vi "TraverseDoAllChannels.vi"(0 "Current Pulses positions for all channels":dbl[](array[numeric]), 1 "Current Pos In Eng units of all channels":dbl[](array[numeric]) format="%.2f", 2 "Counters Reset?":bool, 5 "Backlash Compensation?":bool, 7 "Home":T1, 9 "Mode":T5, 11 "Position Steps":dbl[][](array[numeric]) format="%.2f", 12 "Matched Configurations all Channels In":T2[](array[typedef]) {"Static Drive Configuration"."Indexer Mode  (FSA)" items=["Incremental", "Absolute"]; "Static Drive Configuration"."Buffer at Stop (SSH)" items=["Clear buffer", "Save and Continue"]; "Static Drive Configuration"."Buffer at Limit (SSG)" items=["Clear buffer", "Save and Continue"]; "Static Drive Configuration"."RS232 Echo Control (SSA)" items=["Echo ON", "Echo OFF"]; "Static Drive Configuration"."Reference edge of Home (OSH)" items=["CW", "CCW"]; "Static Drive Configuration"."Encoder Z for Home (OSD)" items=["Don't use", "Enable"]; "Static Drive Configuration"."Home Switch Sense (OSC)" items=["Normally Open", "Normally Closed"]; "Static Drive Configuration"."Home Position (OSB)" items=["Anywhere in Switch", "Edge of Switch"]; "Static Drive Configuration"."Limit Switch Sense (OSA)" items=["Normally Closed", "Normally Open"]; "Static Drive Configuration"."Limit Disable (LD)" items=["Both Enabled", "CW Disabled", "CCW Disabled", "Both Disabled"]; "Static Drive Configuration"."Stall Detect (FSH)" items=["Disable", "Enable"]; "Static Drive Configuration"."OP2 in Deadband (FSG)" items=["Don't Use", "ACTIVATE"]; "Static Drive Configuration"."Stop on Trigger 3 (FSF)" items=["Ignore", "STOP!"]; "Static Drive Configuration"."Activate OP1 on stall (FSE)" items=["Do not Activate", "ACTIVATE!"]; "Static Drive Configuration"."Stop on Stall (FSD)" items=["Continue", "STOP"]; "Static Drive Configuration"."Position Maintenance (FSC)" items=["Disabled", "Enabled"]; "Static Drive Configuration"."Step Mode  (FSB)" items=["Motor", "Encoder"]; "Static Drive Configuration"."Encoder Resolution (ER)" min=1 max=50000; "Static Drive Configuration"."Dead Band Window (DW)" min=0 max=999999999; "Static Drive Configuration"."Dead Band (DB)" min=0 max=999999999; "Static Drive Configuration"."Correction Gain % (CG)" items=["n/a", "12.5", "25", "37.5", "50", "62.5", "75", "87.5", "100"]; "Channel Properties"."Current Pos" format="%.2f"; "Channel Properties"."Backlash/Eng units" format="%.2f"; "Channel Properties"."Pulses/rev" format="%.2f"; "Channel Properties"."Pos Tolerance" format="%.2f"; "Channel Properties"."Pulses/unit" format="%.2f"; "Channel Properties"."Acc. Min" format="%.2f"; "Channel Properties"."Acc. Max" format="%.2f"; "Channel Properties"."Vel. Min" format="%.2f"; "Channel Properties"."Vel. Max" format="%.2f"; "Channel Properties"."Acc. Default" format="%.2f"; "Channel Properties"."Vel. Default" format="%.2f"}, 13 "Last Part of Move?":bool, 14 "Traverse Name":string="EnFlo Tunnel") -> (4 "Achieved Pos In Eng units of all channels":dbl[](array[numeric]) format="%.2f", 6 "Current Pulses positions for all channels Out":dbl[](array[numeric]), 10 "Error String":string, 15 "Matched Configurations Out":T2[](array[typedef]) {"Static Drive Configuration"."Indexer Mode  (FSA)" items=["Incremental", "Absolute"]; "Static Drive Configuration"."Buffer at Stop (SSH)" items=["Clear buffer", "Save and Continue"]; "Static Drive Configuration"."Buffer at Limit (SSG)" items=["Clear buffer", "Save and Continue"]; "Static Drive Configuration"."RS232 Echo Control (SSA)" items=["Echo ON", "Echo OFF"]; "Static Drive Configuration"."Reference edge of Home (OSH)" items=["CW", "CCW"]; "Static Drive Configuration"."Encoder Z for Home (OSD)" items=["Don't use", "Enable"]; "Static Drive Configuration"."Home Switch Sense (OSC)" items=["Normally Open", "Normally Closed"]; "Static Drive Configuration"."Home Position (OSB)" items=["Anywhere in Switch", "Edge of Switch"]; "Static Drive Configuration"."Limit Switch Sense (OSA)" items=["Normally Closed", "Normally Open"]; "Static Drive Configuration"."Limit Disable (LD)" items=["Both Enabled", "CW Disabled", "CCW Disabled", "Both Disabled"]; "Static Drive Configuration"."Stall Detect (FSH)" items=["Disable", "Enable"]; "Static Drive Configuration"."OP2 in Deadband (FSG)" items=["Don't Use", "ACTIVATE"]; "Static Drive Configuration"."Stop on Trigger 3 (FSF)" items=["Ignore", "STOP!"]; "Static Drive Configuration"."Activate OP1 on stall (FSE)" items=["Do not Activate", "ACTIVATE!"]; "Static Drive Configuration"."Stop on Stall (FSD)" items=["Continue", "STOP"]; "Static Drive Configuration"."Position Maintenance (FSC)" items=["Disabled", "Enabled"]; "Static Drive Configuration"."Step Mode  (FSB)" items=["Motor", "Encoder"]; "Static Drive Configuration"."Encoder Resolution (ER)" min=1 max=50000; "Static Drive Configuration"."Dead Band Window (DW)" min=0 max=999999999; "Static Drive Configuration"."Dead Band (DB)" min=0 max=999999999; "Static Drive Configuration"."Correction Gain % (CG)" items=["n/a", "12.5", "25", "37.5", "50", "62.5", "75", "87.5", "100"]; "Channel Properties"."Current Pos" format="%.2f"; "Channel Properties"."Backlash/Eng units" format="%.2f"; "Channel Properties"."Pulses/rev" format="%.2f"; "Channel Properties"."Pos Tolerance" format="%.2f"; "Channel Properties"."Pulses/unit" format="%.2f"; "Channel Properties"."Acc. Min" format="%.2f"; "Channel Properties"."Acc. Max" format="%.2f"; "Channel Properties"."Vel. Min" format="%.2f"; "Channel Properties"."Vel. Max" format="%.2f"; "Channel Properties"."Acc. Default" format="%.2f"; "Channel Properties"."Vel. Default" format="%.2f"})   [LabVIEW 2014]
uses:
  Anemometry/Anemometry Sub Vis/Gen Trav/Trav_mode.ctl
  ~subVIs/AxisConfigCluster.ctl
  ~subVIs/DriveProperties.ctl
  ~subVIs/DriveStaticConfig.ctl
  Anemometry/Anemometry Sub Vis/Controls/Home.ctl
  ~subVIs/DriveGotoCluster.ctl
  ~subVIs/DriveConfigGlobal.vi
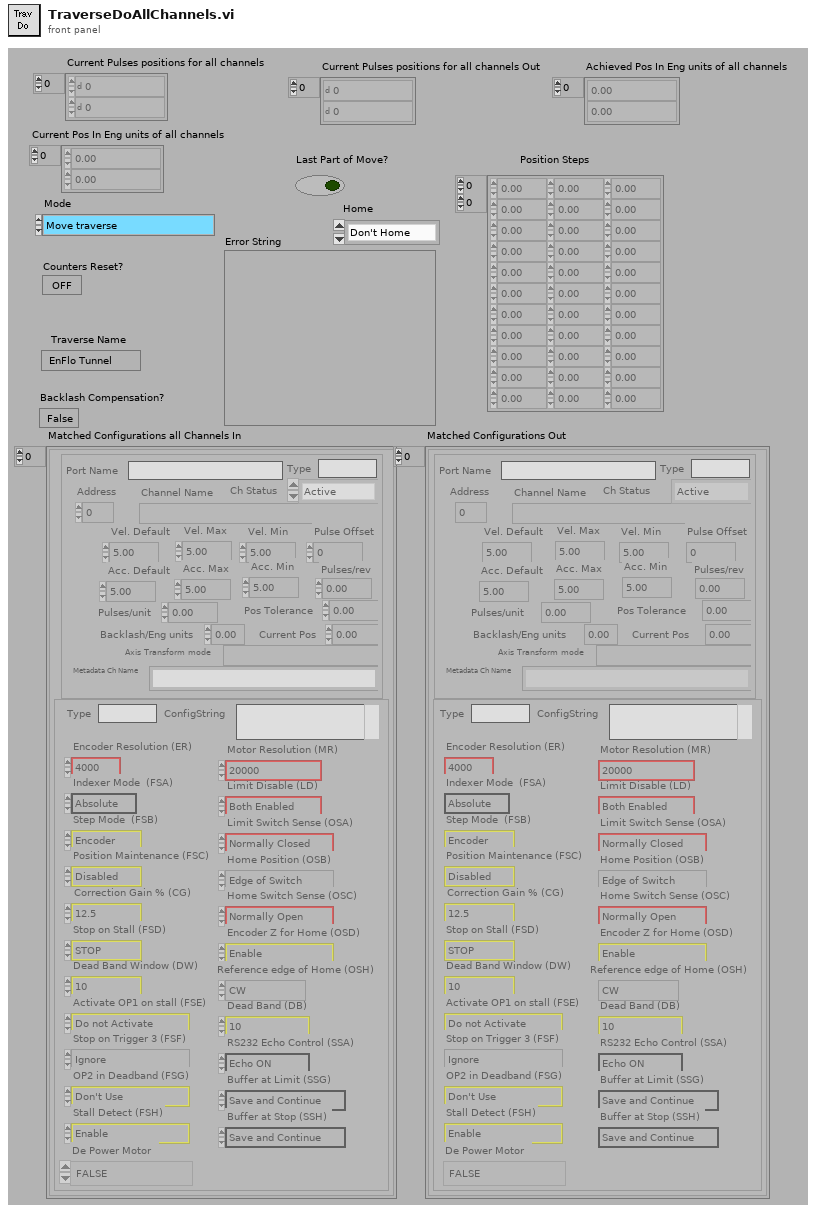
[diagram p1: front panel]
types:
  T1 = typedef "Home.ctl" = enum16{"Don't Home", "Home  +X", "Home  -X", "Home  +Y", "Home  -Y", "Home  +Z", "Home  -Z"}
  T2 = typedef "AxisConfigCluster.ctl" = cluster{"Channel Properties":T3, "Static Drive Configuration":T4}
  T3 = typedef "DriveProperties.ctl" = cluster{"Channel Name":string, "Vel. Default":dbl, "Acc. Default":dbl, "Vel. Max":dbl, "Vel. Min":dbl, "Acc. Max":dbl, "Acc. Min":dbl, "Pulses/unit":dbl, "Address":u8, "Pulse Offset":i32, "Pos Tolerance":dbl, "Pulses/rev":dbl, "Backlash/Eng units":dbl, "Current Pos":dbl, "Ch Status":enum16{"Active", "Offline", "Simulate"}, "Port Name":string, "Axis Transform mode":string, "Metadata Ch Name":string, "Type":string}
  T4 = typedef "DriveStaticConfig.ctl" = cluster{"Correction Gain % (CG)":u16, "Dead Band (DB)":i32, "Dead Band Window (DW)":i32, "Encoder Resolution (ER)":i32, "Step Mode  (FSB)":u16, "Position Maintenance (FSC)":u16, "Stop on Stall (FSD)":u16, "Activate OP1 on stall (FSE)":u16, "Stop on Trigger 3 (FSF)":u16, "OP2 in Deadband (FSG)":u16, "Stall Detect (FSH)":u16, "Limit Disable (LD)":u16, "Motor Resolution (MR)":enum16{"200", "400", "1000", "2000", "4000", "5000", "10000", "12800", "18000", "20000", "21600", "25000", "25400", "25600", "36000", "50000", "278528", "425984", "507904", "614400", "655360", "819200", "1024000"}, "Limit Switch Sense (OSA)":u16, "Home Position (OSB)":u16, "Home Switch Sense (OSC)":u16, "Encoder Z for Home (OSD)":u16, "Reference edge of Home (OSH)":u16, "RS232 Echo Control (SSA)":u16, "Buffer at Limit (SSG)":u16, "Buffer at Stop (SSH)":u16, "Indexer Mode  (FSA)":u16, "Type":string, "ConfigString":string, "De Power Motor":enum16{"TRUE", "FALSE"}}
  T5 = typedef "Trav_mode.ctl" = enum16{"Move traverse", "Read traverse position", "Teach Position"}
  T6 = enum16{"Load setup from excel file", "Save setup to excel file"}
  T7 = typedef "DriveGotoCluster.ctl" = cluster{"Channel name":string, "Go To Position":dbl}
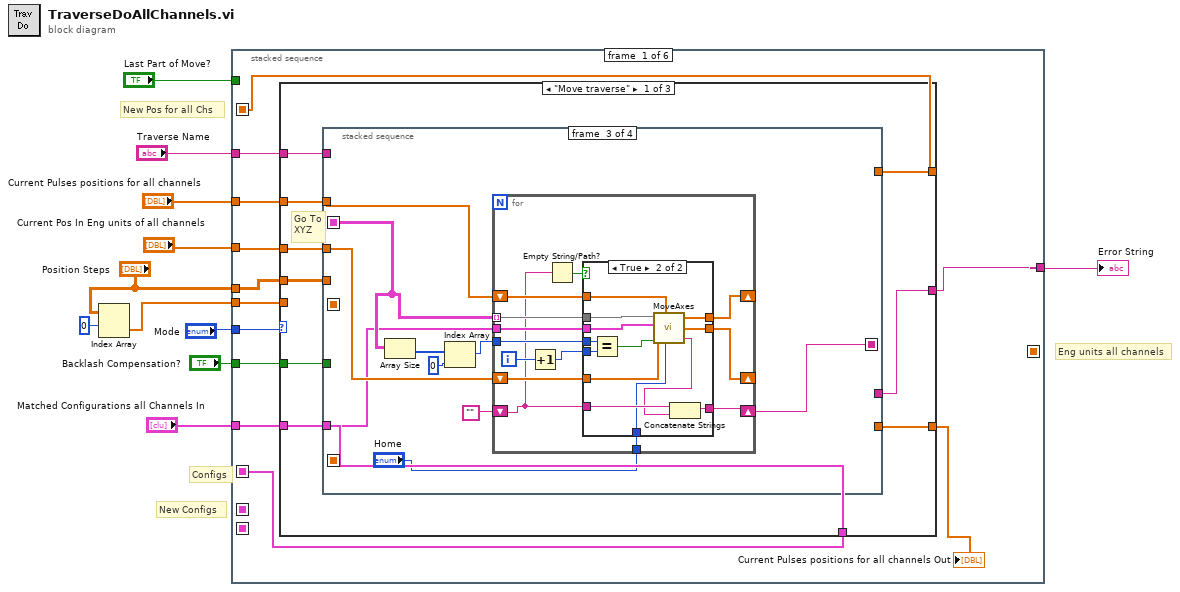
[diagram p0: block diagram]
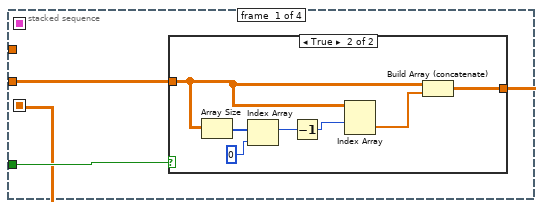
[diagram p2: hidden frame]
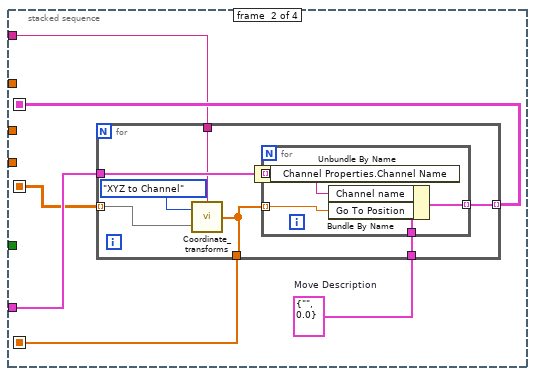
[diagram p4: hidden frame]
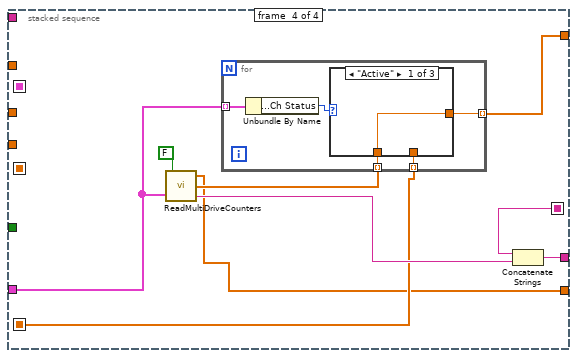
[diagram p6: hidden frame]
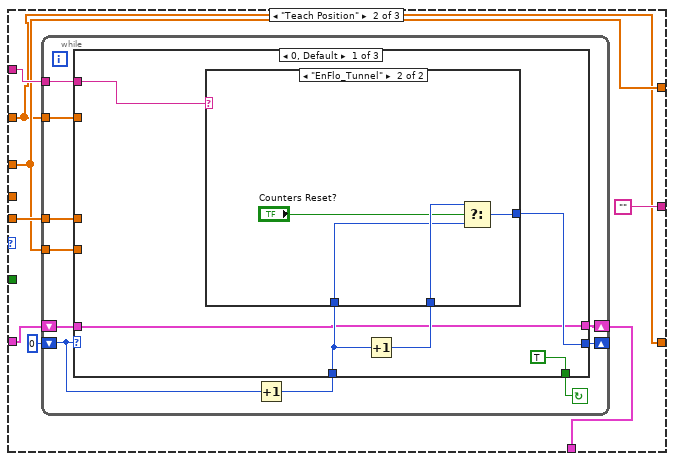
[diagram p9: hidden frame]
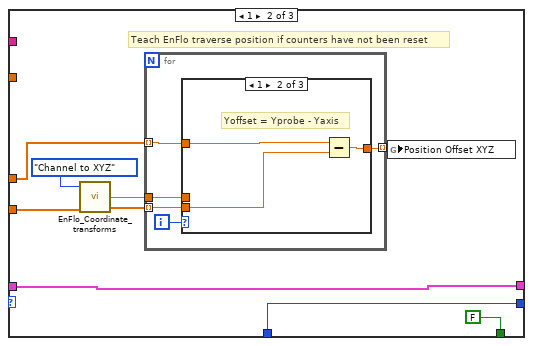
[diagram p11: hidden frame]
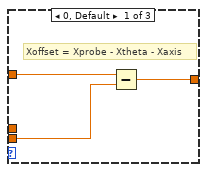
[diagram p12: hidden frame]
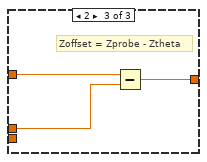
[diagram p13: hidden frame]
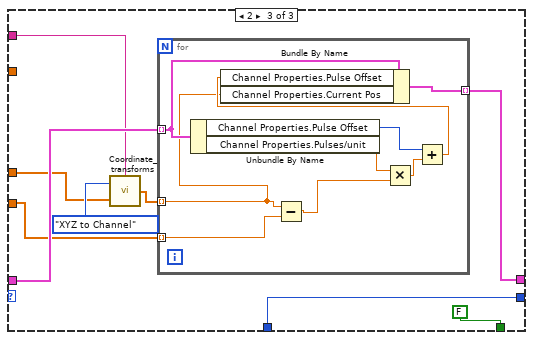
[diagram p14: hidden frame]
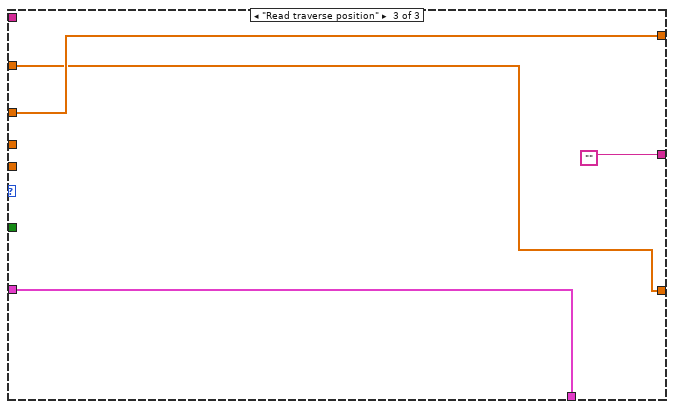
[diagram p15: hidden frame]
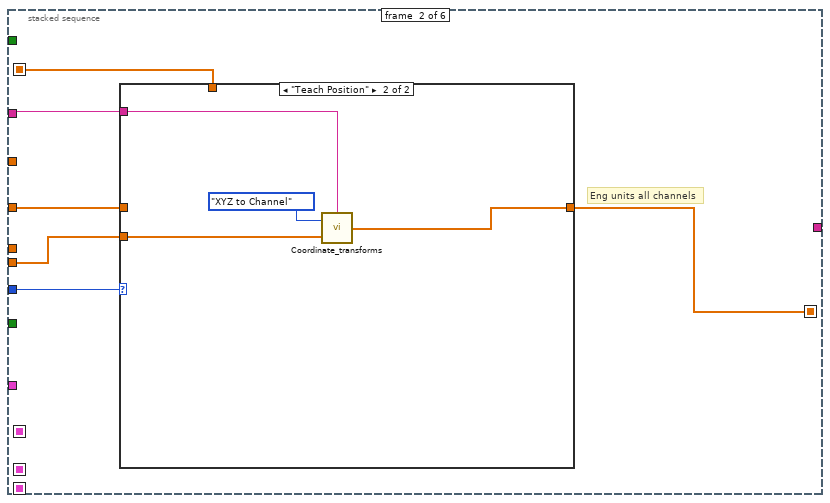
[diagram p16: hidden frame]
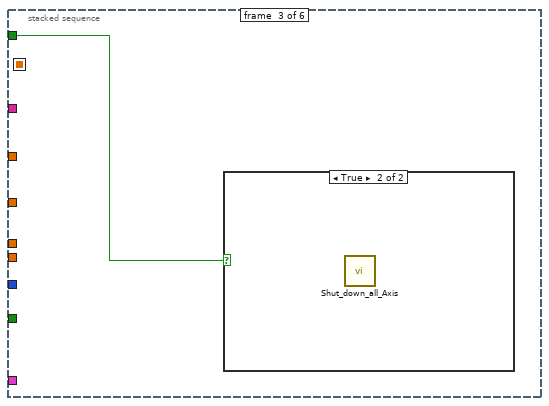
[diagram p18: hidden frame]
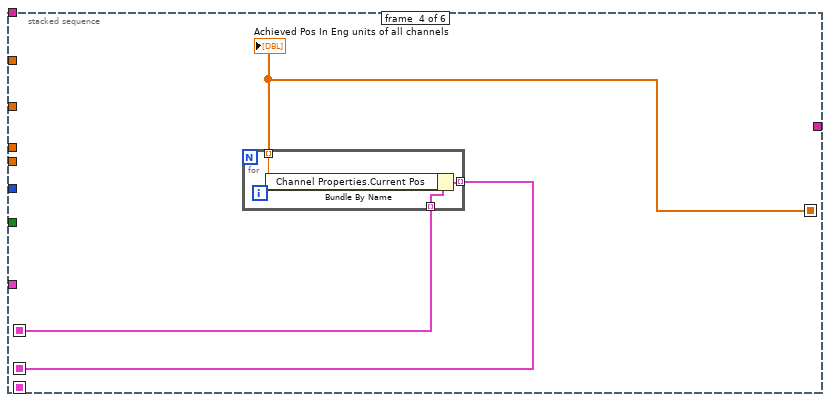
[diagram p20: hidden frame]
diagram:
  # "New Pos for all Chs"
  # "Eng units all channels"
  # "New Configs"
  # "Configs"
  n1 = Index Array(array="Position Steps", index (row)=0 ("Index")) -> (element=w2:dbl[])  [unwired: 1 in]
  n2 = stacked-sequence {
    seq-local: [_ w195 _ _ _ _] -> [_ _ _ w204 _ _]
    seq-local: [w22 _ _ _ _ _] -> [_ _ _ w206 _ _]
    seq-local: [_ _ _ w205 _ _] -> [_ _ _ _ w213 _]
    seq-local: [w13 _ _ _ _ _] -> [_ w192 _ _ _ _]
    seq-local: [_ _ _ _ w211 _] -> [_ _ _ _ _ w220]
    tunnel: "Mode" -> [w23 w196 _ _ _ w221]
    tunnel: "Current Pos In Eng units of all channels" -> [w20 w197 _ _ _ _]
    tunnel: "Matched Configurations all Channels In" -> [w21 _ _ _ _ _]
    tunnel: "Current Pulses positions for all channels" -> [w19 _ _ _ _ _]
    tunnel: [w18 _ _ _ _ _] -> w7
    tunnel: "Traverse Name" -> [w17 w194 _ _ w212 w219]
    tunnel: "Position Steps" -> [w16 _ _ _ _ _]
    tunnel: "Backlash Compensation?" -> [w15 _ _ _ _ _]
    tunnel: w2 -> [w14 w193 _ _ _ _]
    tunnel: "Last Part of Move?" -> [_ _ w203 _ w210 _]
    frame #0 {
      n3 = case shown="\"Move traverse\"" w23 {
        tunnel: [w32 w122 w191] -> w22
        tunnel: w21 -> [w32 w123 w191]
        tunnel: w20 -> [w30 w119 w189]
        tunnel: w19 -> [w31 w118 w188]
        tunnel: [w29 "" ""] -> w18
        tunnel: w17 -> [w27 w124 _]
        tunnel: w16 -> [w28 _ _]
        tunnel: w15 -> [w26 _ _]
        tunnel: w14 -> [_ w120 _]
        tunnel: [w25 w119 w189] -> w13
        tunnel: [w24 w118 w188] -> w12
        frame "Move traverse" {
          # "Go To\nXYZ"
          n4 = stacked-sequence {
            seq-local: [_ w47 _ _] -> [_ _ w65 _]
            seq-local: [w34 _ _ _] -> [_ w46 _ _]
            seq-local: [_ _ w63 _] -> [_ _ _ w108]
            seq-local: [_ w44 _ _] -> [_ _ _ w102]
            tunnel: w32 -> [_ w48 w64 w105]
            tunnel: w31 -> [_ _ w71 _]
            tunnel: w30 -> [_ _ w70 _]
            tunnel: [_ _ _ w106] -> w29
            tunnel: w28 -> [w33 _ _ _]
            tunnel: w27 -> [_ w45 _ _]
            tunnel: w26 -> [w35 _ _ _]
            tunnel: [_ _ _ w104] -> w25
            tunnel: [_ _ _ w101] -> w24
            frame #0 {
              n5 = case shown="True" w35 {
                tunnel: w33 -> [w36 w38]
                tunnel: [w36 w37] -> w34
                frame False {
                }
                frame True {
                  n6 = Array Size(array=w38) -> (size(s)=w43:i32[])
                  n7 = Index Array(array=w43, index=0 ("Index")) -> (element=w41:i32)
                  n8 = Decrement(x=w41) -> (x-1=w40:i32)
                  n9 = Index Array(array=w38, index (row)=w40) -> (element=w39:dbl[])  [unwired: 1 in]
                  n10 = Build Array (concatenate)(w38, w39) -> (w37:dbl[][])
                }
              }
            }
            frame #1 {
              w49 = T7 {"Channel name"="", "Go To Position"=0.0}  # Move Description
              n11 = for {
                tunnel: w49 -> [w56]
                tunnel: w48 -> [w55]
                tunnel: [w54] -> w47 mode=indexing
                tunnel: w46 -> [w51] mode=indexing
                tunnel: w45 -> [w52]
                tunnel: [w50] -> w44
                n12 = call "Coordinate_transforms.vi"("Traverse Name"=w52, "Input"=w51, "Mode"=enum16{"XYZ to Channel", "Channel to XYZ"}."XYZ to Channel") -> ("Output"=w50:dbl[])
                n13 = for {
                  tunnel: w50 -> [w61] mode=indexing
                  tunnel: [w60] -> w54 mode=indexing
                  tunnel: w55 -> [w58] mode=indexing
                  tunnel: w56 -> [w57]
                  n14 = Unbundle By Name(w58) -> ("Channel Properties.Channel Name"=w59:string)
                  n15 = Bundle By Name(cluster=w57, "Channel name"=w59, "Go To Position"=w61) -> (w60:T7)
                }
              }
            }
            frame #2 {
              n16 = Array Size(array=w65) -> (size(s)=w68:i32[])
              n17 = Index Array(array=w68, index=0 ("Index")) -> (element=w66:i32)
              n18 = for {
                tunnel: w65 -> [w84] mode=indexing
                tunnel: w64 -> [w83]
                shift-right: [w80] -> _
                shift-left: w71 -> [w79]
                shift-right: [w81] -> _
                shift-left: w70 -> [w82]
                tunnel: w66 -> [w76]
                shift-right: [w75] -> w63
                shift-left: "" -> [w74]
                tunnel: "Home" -> [w72]
                i -> [w78]
                n19 = Increment(x=w78) -> (x+1=w77:i32)
                n20 = Empty String/Path?(string/path=w74) -> (empty?=w73:bool)
                n21 = case shown="True" w73 {
                  tunnel: w84 -> [_ w100]
                  tunnel: w83 -> [_ w99]
                  tunnel: w82 -> [w86 w98]
                  tunnel: [w86 w97] -> w81
                  tunnel: [w87 w96] -> w80
                  tunnel: w79 -> [w87 w95]
                  tunnel: w77 -> [_ w94]
                  tunnel: w76 -> [_ w93]
                  tunnel: [w85 w90] -> w75
                  tunnel: w74 -> [w85 w92]
                  tunnel: w72 -> [_ w88]
                  frame False {
                  }
                  frame True {
                    n22 = Equal?(x=w93, y=w94) -> (x = y?=w89:bool)
                    n23 = call "MoveAxes.vi"("GoTo Array (Eng units all channels)"=w100, "Current Pulses In"=w95, "Matched Configurations"=w99, "Current Pos In"=w98, "Home"=w88, "Final move"=w89) -> ("Current Pulses Out"=w96:dbl[], "Current Pos Out"=w97:dbl[], "Error String"=w91:string)
                    n24 = Concatenate Strings(w92, w91) -> (w90:string)
                  }
                }
              }
            }
            frame #3 {
              n25 = call "ReadMultiDriveCounters.vi"("Recheck if Moved?"=FALSE, "Matched Configurations"=w105) -> ("Pulses"=w101:dbl[], "Eng units"=w103:dbl[], "Error String"=w107:string)
              n26 = for {
                tunnel: w105 -> [w114] mode=indexing
                tunnel: [w112] -> w104 mode=indexing
                tunnel: w103 -> [w111] mode=indexing
                tunnel: w102 -> [w110] mode=indexing
                n27 = Unbundle By Name(w114) -> ("Channel Properties.Ch Status"=w113:enum16{"Active", "Offline", "Simulate"})
                n28 = case shown="\"Active\"" w113 {
                  tunnel: [w115 w116 w117] -> w112
                  tunnel: w111 -> [w115 _ w117]
                  tunnel: w110 -> [_ w116 _]
                  frame "Active" {
                  }
                  frame "Simulate" {
                  }
                  frame "Offline" {
                  }
                }
              }
              n29 = Concatenate Strings(w108, w107) -> (w106:string)
            }
          }
        }
        frame "Teach Position" {
          n30 = while {
            tunnel: w120 -> [w126]
            shift-left: w123 -> [w128]
            shift-right: [w127] -> w122
            tunnel: w119 -> [w129]
            tunnel: w118 -> [w130]
            tunnel: w124 -> [w131]
            shift-left: 0 -> [w135]
            shift-right: [w132] -> _
            stop <- w134 continue-if-true
            n31 = Increment(x=w135) -> (x+1=w133:i32)
            n32 = case shown="0, Default" w135 {
              tunnel: [TRUE FALSE FALSE] -> w134
              tunnel: w133 -> [w138 w149 w178]
              tunnel: [w139 w149 w178] -> w132
              tunnel: w131 -> [w140 _ w171]
              tunnel: w130 -> [_ _ _]
              tunnel: w129 -> [_ w150 w172]
              tunnel: w128 -> [w136 w148 w176]
              tunnel: [w136 w148 w175] -> w127
              tunnel: w126 -> [_ w147 w170]
              frame 0, Default {
                n33 = Increment(x=w138) -> (x+1=w137:i32)
                n34 = case shown="\"EnFlo_Tunnel\"" w140 {
                  tunnel: [w142 w146] -> w139
                  tunnel: w138 -> [_ w144]
                  tunnel: w137 -> [w142 w145]
                  frame "A_Tunnel", Default {
                  }
                  frame "EnFlo_Tunnel" {
                    n35 = Select(t=w145, s="Counters Reset?", f=w144) -> (s? t:f=w146:i32)
                  }
                }
              }
              frame 1 {
                # "Teach EnFlo traverse position if counters have not been reset"
                n36 = call "EnFlo_Coordinate_transforms.vi"("Input"=w150, "Mode"=enum16{"XYZ to Channel", "Channel to XYZ"}."Channel to XYZ") -> ("Output"=w153:dbl[], "Z theta"=w152:dbl)  [unwired: 2 out]
                n37 = for {
                  tunnel: w147 -> [w159] mode=indexing
                  tunnel: w153 -> [w158] mode=indexing
                  tunnel: [w157] -> w154 mode=indexing
                  tunnel: w152 -> [w156]
                  i -> [w160]
                  n38 = case shown="1" w160 {
                    tunnel: w159 -> [w163 w166 w169]
                    tunnel: w158 -> [w162 w165 _]
                    tunnel: [w161 w164 w167] -> w157
                    tunnel: w156 -> [_ _ w168]
                    frame 0, Default {
                      # "Xoffset = Xprobe - Xtheta - Xaxis"
                      n39 = Subtract(x=w163, y=w162) -> (x-y=w161:dbl)
                    }
                    frame 1 {
                      # "Yoffset = Yprobe - Yaxis"
                      n40 = Subtract(x=w166, y=w165) -> (x-y=w164:dbl)
                    }
                    frame 2 {
                      # "Zoffset = Zprobe - Ztheta"
                      n41 = Subtract(x=w169, y=w168) -> (x-y=w167:dbl)
                    }
                  }
                }
                n42 = global write "DriveConfigGlobal.vi" "Position Offset XYZ"(w154) -> ()
              }
              frame 2 {
                n43 = call "Coordinate_transforms.vi"("Traverse Name"=w171, "Input"=w170, "Mode"=enum16{"XYZ to Channel", "Channel to XYZ"}."XYZ to Channel") -> ("Output"=w173:dbl[])
                n44 = for {
                  tunnel: w176 -> [w187] mode=indexing
                  tunnel: [w185] -> w175 mode=indexing
                  tunnel: w172 -> [w183] mode=indexing
                  tunnel: w173 -> [w179] mode=indexing
                  n45 = Unbundle By Name(w187) -> ("Channel Properties.Pulse Offset"=w184:i32, "Channel Properties.Pulses/unit"=w182:dbl)
                  n46 = Subtract(x=w179, y=w183) -> (x-y=w180:dbl)
                  n47 = Multiply(x=w182, y=w180) -> (x*y=w181:dbl)
                  n48 = Add(x=w184, y=w181) -> (x+y=w186:dbl)
                  n49 = Bundle By Name(cluster=w187, "Channel Properties.Pulse Offset"=w186, "Channel Properties.Current Pos"=w179) -> (w185:T2)
                }
              }
            }
          }
        }
        frame "Read traverse position" {
        }
      }
      "Current Pulses positions for all channels Out" <- w12
    }
    frame #1 {
      # "Eng units all channels"
      n50 = case shown="\"Teach Position\"" w196 {
        tunnel: w197 -> [_ _]
        tunnel: [w198 w201] -> w195
        tunnel: w194 -> [_ w200]
        tunnel: w193 -> [_ w199]
        tunnel: w192 -> [w198 _]
        frame "Move traverse", Default {
        }
        frame "Teach Position" {
          n51 = call "Coordinate_transforms.vi"("Traverse Name"=w200, "Input"=w199, "Mode"=enum16{"XYZ to Channel", "Channel to XYZ"}."XYZ to Channel") -> ("Output"=w201:dbl[])
        }
      }
    }
    frame #2 {
      n52 = case shown="True" w203 {
        frame False {
        }
        frame True {
          n53 = call "Shut_down_all_Axis.vi"() -> ()  [unwired: 1 out]
        }
      }
    }
    frame #3 {
      n54 = for {
        tunnel: [w209] -> w205 mode=indexing
        tunnel: w206 -> [w208] mode=indexing
        tunnel: w204 -> [w207] mode=indexing
        n55 = Bundle By Name(cluster=w208, "Channel Properties.Current Pos"=w207) -> (w209:T2)
      }
      "Achieved Pos In Eng units of all channels" <- w204
    }
    frame #4 {
      n56 = case shown="False" w210 {
        tunnel: w213 -> [w214 w217]
        tunnel: w212 -> [_ w216]
        tunnel: [w214 w215] -> w211
        frame False {
        }
        frame True {
          n57 = call "Read_Write_Trav_position.vi"("Matched Configurations In"=w217, "Mode"=T6."Save setup to excel file", "Traverse Name"=w216) -> ("Matched Configurations Out"=w215:T2[])  [unwired: 1 out]
        }
      }
      "Matched Configurations Out" <- w211
    }
    frame #5 {
      n58 = case shown="\"Teach Position\"" w221 {
        tunnel: w220 -> [_ w223]
        tunnel: w219 -> [_ w222]
        frame "Move traverse", Default {
        }
        frame "Teach Position" {
          n59 = stacked-sequence {
            tunnel: w223 -> [w226 _]
            tunnel: w222 -> [_ w236]
            frame #0 {
              n60 = global read "DriveConfigGlobal.vi" "Configurations"() -> (w225:T2[])
              n61 = for {
                tunnel: w225 -> [w235] mode=indexing
                tunnel: [w234] -> w227 mode=indexing
                n62 = Unbundle By Name(w235) -> ("Channel Properties.Channel Name"=w234:string)
              }
              n63 = for {
                tunnel: w227 -> [w233]
                tunnel: w226 -> [w228] mode=indexing
                shift-right: [w230] -> w224
                shift-left: w225 -> [w231]
                n64 = Unbundle By Name(w228) -> ("Channel Properties.Channel Name"=w232:string)
                n65 = Search 1D Array(1D array=w233, element=w232) -> (index of element=w229:i32)  [unwired: 1 out]
                n66 = Replace Array Subset(array=w231, new element=w228, index=w229) -> (w230:T2[])
              }
              n67 = global write "DriveConfigGlobal.vi" "Configurations"(w224) -> ()
            }
            frame #1 {
              n68 = call "Read_Write_Trav_Config.vi"("Traverse Name"=w236, "Mode"=T6."Save setup to excel file") -> ()  [unwired: 1 out]
            }
          }
        }
      }
    }
  }
  "Error String" <- w7
